vi "Get Section.vi"(11 "Supported Objects in":refnum<class "Supported Objects.lvclass">) -> (2 "Section":string, 3 "Supported Objects out":refnum<class "Supported Objects.lvclass">)   [LabVIEW 2024, in "Electronic Datasheet.lvlib" / "Supported Objects.lvclass"]
uses:
  Supported Objects.lvclass
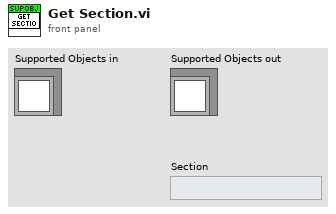
[diagram p1: front panel]
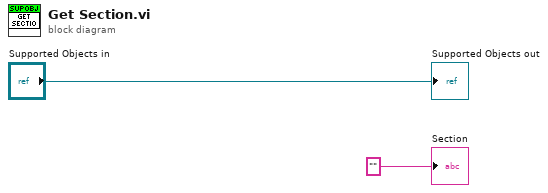
[diagram p0: block diagram]
diagram:
  "Supported Objects out" <- "Supported Objects in"
  "Section" <- "" ("Section")
